vi "CUST Get Digital Configuration.vi"(9 "digitalIndex":i32, 10 "pmuIndex":i32, 11 "pseudoPdcId":i32) -> (0 "function return":i32, 2 "name out":string, 3 "digitalCfg out":cluster{"normalBit":u8, "isValidBit":u8})   [LabVIEW 2013, in "C37118-DLL.lvlib"]
doc: "STRONGRIDIEEEC37118DLL_API int __cdecl getDigitalConfigLabview(noArraysDigitalConfig* digitalCfg, char* name, int32_t pseudoPdcId, int32_t pmuIndex, int32_t digitalIndex );"
uses:
  C37118-DLL.lvlib
  Auto Generated/StrongridDLL.dll
panel:
  in  "name":string
  in  "digitalCfg":cluster{"normalBit":u8, "isValidBit":u8}
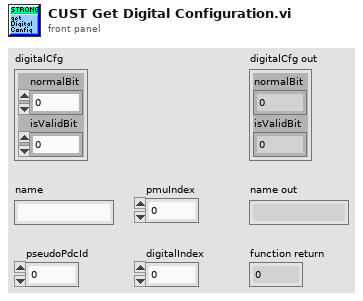
[diagram p1: front panel]
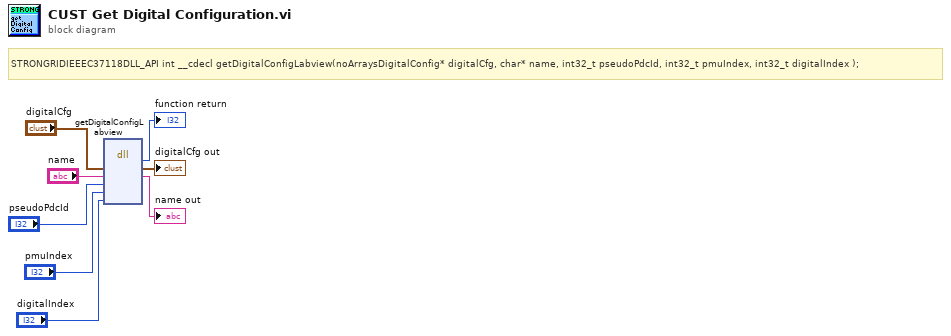
[diagram p0: block diagram]
diagram:
  # "STRONGRIDIEEEC37118DLL_API int __cdecl getDigitalConfigLabview(noArraysDigitalConfig* digitalCfg, char* name, int32_t pseudoPdcId, int32_t pmuIndex, int32_t digitalIndex );"
  n1 = dll-call lib="C:/Prevas/Projects/statnett/AFS171 Statnett PMU Reference Library/afs171.sw/LabVIEW PRL Library LV2013/c37118-dll/labview/vi/Auto Generated/StrongridDLL.*" fn="getDigitalConfigLabview"("digitalCfg"="digitalCfg", "name"="name", "pseudoPdcId"="pseudoPdcId", "pmuIndex"="pmuIndex", "digitalIndex"="digitalIndex") -> (→"function return":i32, "digitalCfg"=→"digitalCfg out":cluster{"normalBit":u8, "isValidBit":u8}, "name"=→"name out":string)  [unwired: 6 in, 2 out]
